vi "Read Lockin.vi"(8 "error in (no error)":errorcluster, 11 "Software Lock-in in":refnum<class "Software Lock-in.lvclass">) -> (0 "error out":errorcluster, 2 "Lockin parameters":T1={"Frequency"=0.0, "Phase"=0.0, "Syncronous"=FALSE, "Points per sine wave"=0, "DDS"=FALSE, "Frequency word"=0, "Phase word"=0, "DDS modulus"=15120, "DDS clock"=125000000.0} {"DDS clock" format="%_17pHz"; "DDS modulus" format="0x%x (%d)"; "Phase" format="%#_gdeg"; "Frequency" format="%_17pHz"}, 3 "Software Lock-in out":refnum<class "Software Lock-in.lvclass">)   [LabVIEW 2020]
uses:
  Software Lock-in.lvclass
  Lockin Parameters.ctl
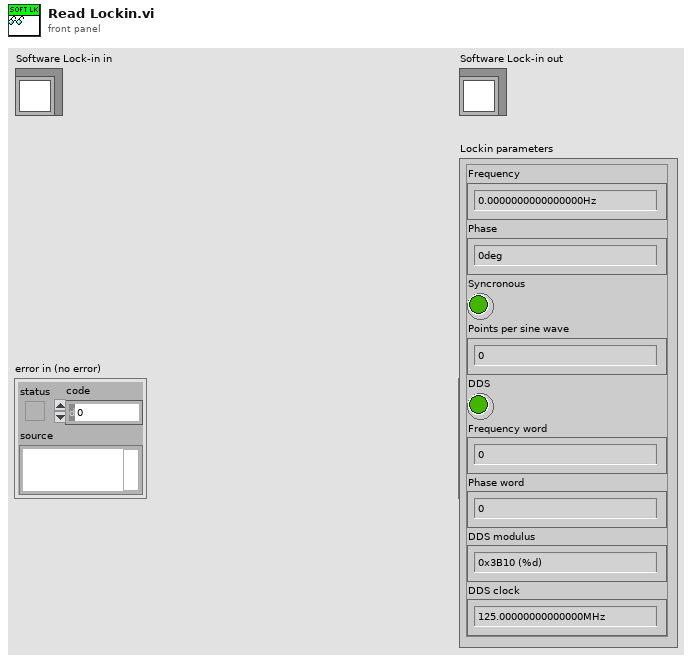
[diagram p1: front panel]
types:
  T1 = typedef "Lockin Parameters.ctl" = cluster{"Frequency":dbl, "Phase":dbl, "Syncronous":bool, "Points per sine wave":i32, "DDS":bool, "Frequency word":u32, "Phase word":u32, "DDS modulus":i64, "DDS clock":dbl}
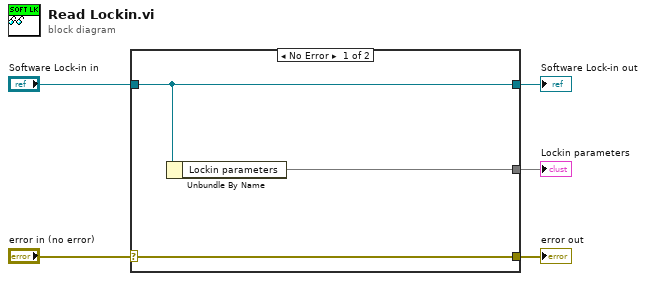
[diagram p0: block diagram]
diagram:
  n1 = case shown="No Error" "error in (no error)" {
    selector: "error in (no error)" -> [w8 w9]
    tunnel: [w8 w9] -> w4
    tunnel: [w7 w10] -> w2
    tunnel: "Software Lock-in in" -> [w7 w10]
    tunnel: [w6 _] -> w1
    frame No Error {
      n2 = Unbundle By Name(w7) -> ("Lockin parameters"=w6)
    }
    frame Error {
    }
  }
  "error out" <- w4
  "Software Lock-in out" <- w2
  "Lockin parameters" <- w1
